vi "MATLAB_helper.vi"(8 "error in (no error)":errorcluster, 11 "Path":path) -> (0 "error out":errorcluster, 2 "XY Graph":cluster{"Array":dbl[], "Array":dbl[]}(graph), 3 "Array":dbl[][](array[numeric]))   [LabVIEW 2017]
uses:
  D:/Jichen/labview/Find_phase_offset_amplitude_function/for_testing/Find_phase_offset_amplitude_functionNative.dll
  Find_phase_offset_amplitude_function/for_testing/Find_phase_offset_amplitude_functionNative.dll
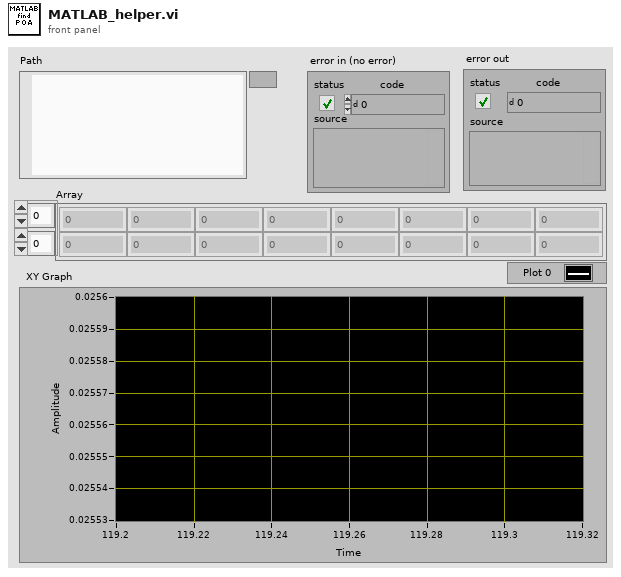
[diagram p1: front panel]
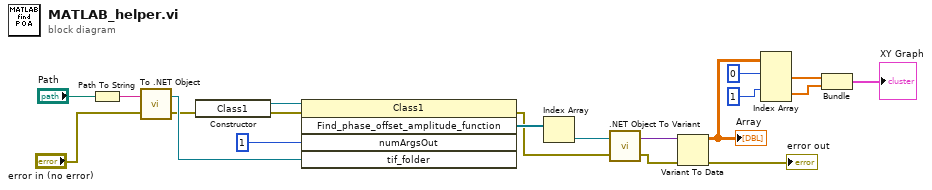
[diagram p0: block diagram]
diagram:
  n1 = Path To String(path="Path") -> (string=w18:string)
  n2 = call <vilib>:"To .NET Object.vi"("error in (no error)"="error in (no error)", "anything"=w18) -> ("error out"=w16:errorcluster, ".NET object"=w17:refnum<k24>)
  n3 = constructor class="Class1"(error in=w16) -> (reference out=w20:refnum<k24>, error out=w15:errorcluster)  [unwired: 2 in, 1 out]
  n4 = invoke class="Class1" method="Find_phase_offset_amplitude_function"(reference=w20, error in=w15, "numArgsOut"=1, "tif_folder"=w17) -> (error out=w12:errorcluster, "Find_phase_offset_amplitude_function"=w14:refnum<k24>[])  [unwired: 1 in, 3 out]
  n5 = Index Array(array=w14) -> (element=w13:refnum<k24>)  [unwired: 1 in]
  n6 = call <vilib>:".NET Object To Variant.vi"("error in (no error)"=w12, ".NET object"=w13) -> ("error out"=w10:errorcluster, "variant"=w11:variant)
  n7 = Variant To Data(error in=w10, Variant=w11) -> (data=w6:dbl[][], error out=→"error out":errorcluster)  [unwired: 1 in]
  "Array" <- w6
  n8 = Index Array(array=w6, index (row) #1=0, index (row) #2=1) -> (element #1=w5:dbl[], element #2=w4:dbl[])  [unwired: 2 in]
  n9 = Bundle("Array"=w5, "Array"=w4) -> (→"XY Graph":cluster{"Array":dbl[], "Array":dbl[]})  [unwired: 1 in]
